vi "Ping.vi"(4 "error in (no error)":errorcluster, 5 "PingQty":i32=10, 6 "timeout (100ms)":i32=100, 7 "hostNameOrAddress":string="192.168.0.100") -> (0 "error out":errorcluster, 1 "Successful Pings":i32=10, 2 "Unsuccessful Pings":i32, 3 "Status":i32(ring) items=["Success"=0, "DestinationNetworkUnreachable"=11002, "DestinationHostUnreachable"=11003, "DestinationProhibited, DestinationProtocolUnreachable"=11004, "DestinationPortUnreachable"=11005, "NoResources"=11006, "BadOption"=11007, "HardwareError"=11008, "PacketTooBig"=11009, "TimedOut"=11010, "BadRoute"=11012, "TtlExpired"=11013, "TtlReassemblyTimeExceeded"=11014, "ParameterProblem"=11015, "SourceQuench"=11016, "BadDestination"=11018, "DestinationUnreachable"=11040, "TimeExceeded"=11041, "BadHeader"=11042, "UnrecognizedNextHeader"=11043, "IcmpError"=11044, "DestinationScopeMismatch"=11045, "Unknown"=-1])   [LabVIEW 2013]
panel:
  out "Pings total":i32=10
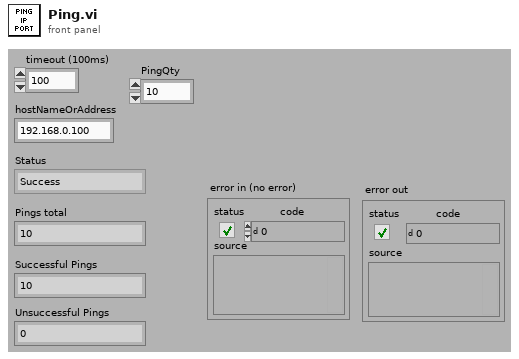
[diagram p1: front panel]
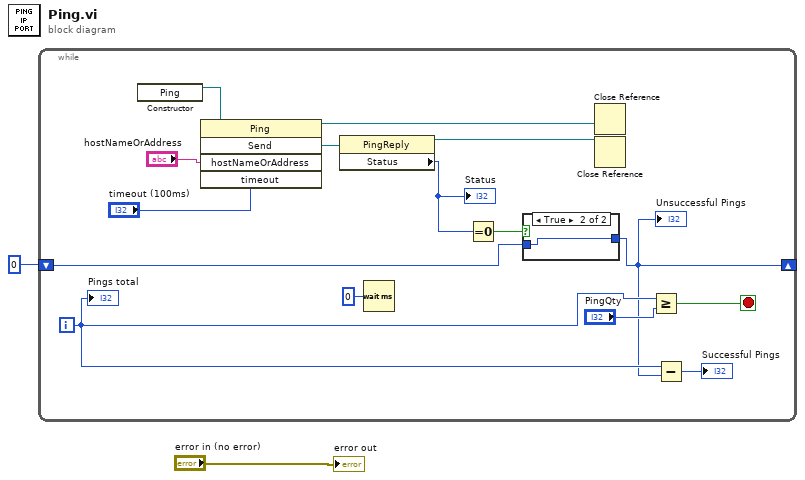
[diagram p0: block diagram]
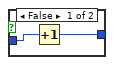
[diagram p2: hidden frame]
diagram:
  n1 = while {
    shift-right: [w3] -> _
    shift-left: u64 0 -> [w12]
    i -> [w4]
    stop <- w7 stop-if-true
    n2 = constructor class="Ping"() -> (reference out=w14:refnum<k24>)  [unwired: 3 in, 2 out]
    n3 = invoke class="Ping" method="Send"(reference=w14, "hostNameOrAddress"="hostNameOrAddress", "timeout"="timeout (100ms)") -> (reference out=w8:refnum<k24>, "Send"=w16:refnum<k24>)  [unwired: 2 in, 3 out]
    n4 = property class="PingReply"(reference=w16) -> (reference out=w9:refnum<k24>, "Status"=w13:i32)  [unwired: 1 in, 1 out]
    "Status" <- w13
    n5 = Wait (ms)(milliseconds to wait=u32 0 ("Zu wartende ms")) -> ()  [unwired: 1 out]
    n6 = Equal To 0?(x=w13) -> (x = 0?=w11:bool)
    n7 = case shown="True" w11 {
      tunnel: w12 -> [w19 w20]
      tunnel: [w18 w20] -> w3
      frame False {
        n8 = Increment(x=w19) -> (x+1=w18:u64)
      }
      frame True {
      }
    }
    "Unsuccessful Pings" <- w3
    n9 = Close Reference(reference=w8) -> ()  [unwired: 1 in, 1 out]
    n10 = Close Reference(reference=w9) -> ()  [unwired: 1 in, 1 out]
    n11 = Greater Or Equal?(x=w4, y="PingQty") -> (x >= y?=w7:bool)
    n12 = Subtract(x=w4, y=w3) -> (x-y=→"Successful Pings":u64)
    "Pings total" <- w4
  }
  "error out" <- "error in (no error)"
